vi "Save Msg.vi"(3 "Saved?":bool, 7 "RFID":string, 12 "RESULT":string) -> (8 "Message":string)   [LabVIEW 2020]
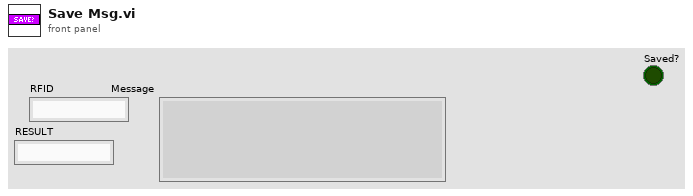
[diagram p1: front panel]
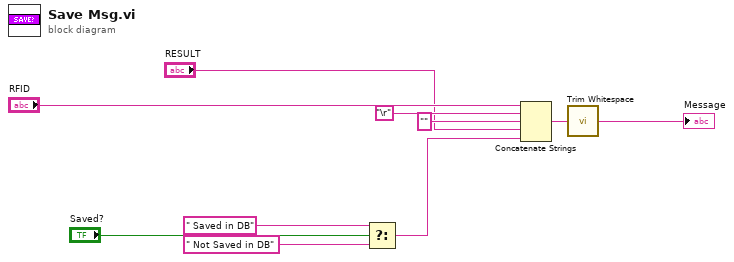
[diagram p0: block diagram]
diagram:
  n1 = Select(t=" Saved in DB" ("Continuty Station Remarks"), s="Saved?", f=" Not Saved in DB" ("Continuty Station Remarks")) -> (s? t:f=w2:string)
  n2 = Concatenate Strings("RFID", "\r", "" ("string"), "RESULT", w2) -> (w8:string)
  n3 = call <vilib>:"Trim Whitespace.vi"("string"=w8) -> ("trimmed string"=→"Message":string)  [unwired: 1 in]
